vi "Connection Check.vi"(0 "Queue in":refnum<queue>, 1 "Producer State In":string, 2 "error in":errorcluster, 3 "error in (no error)":errorcluster, 4 "Connected":bool=TRUE, 5 "Receiving Data":bool=TRUE) -> (7 "Queue out":refnum<queue>, 8 "Producer State Out":string, 10 "error out":errorcluster)   [LabVIEW 2019]
uses:
  MessageFormat1.ctl
  <vilib>/Utility/error.llb/Error Cluster From Error Code.vi
  <vilib>/ErrorRing/Error Ring.xnode
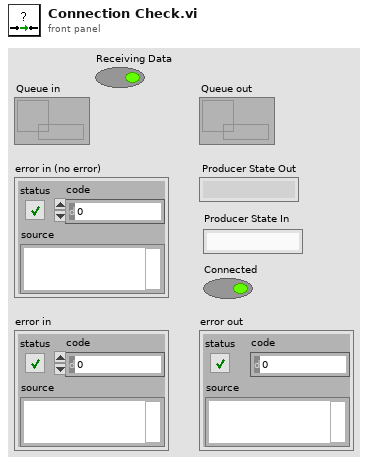
[diagram p1: front panel]
types:
  T1 = typedef "MessageFormat1.ctl" = cluster{"Consumer State":string, "RxData":string, "error constant":errorcluster, "Connected":bool, "Receiving Data":bool, "Producer State ":string}
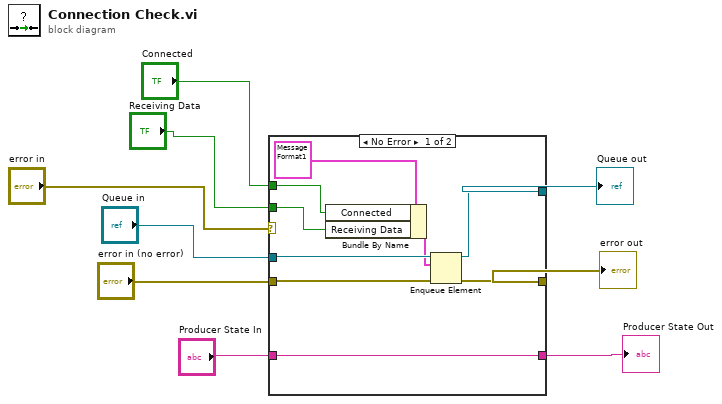
[diagram p0: block diagram]
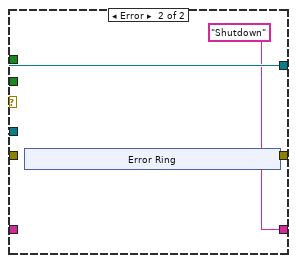
[diagram p2: hidden frame]
diagram:
  n1 = case shown="No Error" "error in" {
    tunnel: "error in (no error)" -> [w18 _]
    tunnel: "Queue in" -> [w17 w21]
    tunnel: [w15 w21] -> w6
    tunnel: [w13 w20] -> w8
    tunnel: [w12 "Shutdown" ("f")] -> w9
    tunnel: "Producer State In" -> [w12 _]
    tunnel: "Connected" -> [w11 _]
    tunnel: "Receiving Data" -> [w10 _]
    frame No Error {
      n2 = Bundle By Name(cluster=T1 {"Consumer State"="Consumer State", "RxData"="Received Data", "error constant"={"status"=FALSE, "code"=0, "source"=""}, "Connected"=FALSE, "Receiving Data"=FALSE, "Producer State "="Consumer State"} ("Queue Definition"), "Connected"=w11, "Receiving Data"=w10) -> (w14:T1)
      n3 = Enqueue Element(queue=w17, element=w14, error in (no error)=w18) -> (queue out=w15:refnum<queue>, error out=w13:errorcluster)  [unwired: 1 in, 1 out]
    }
    frame Error {
      n4 = xnode "Error Ring"() -> ("error out"=w20:errorcluster)
    }
  }
  "Producer State Out" <- w9
  "error out" <- w8
  "Queue out" <- w6
